vi "ДЗ Файлы.vi"() -> ()   [LabVIEW 2021]
panel:
  out "text":string
  out "XY Graph":cluster{i32[], dbl[]}[](graph)
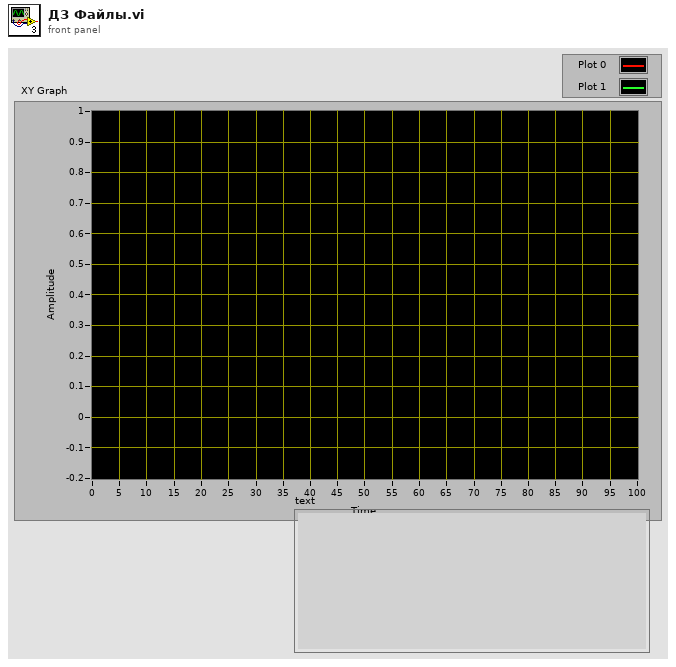
[diagram p1: front panel]
types:
  T1 = enum16{"open", "replace", "create", "open or create", "replace or create", "replace or create with confirmation"}
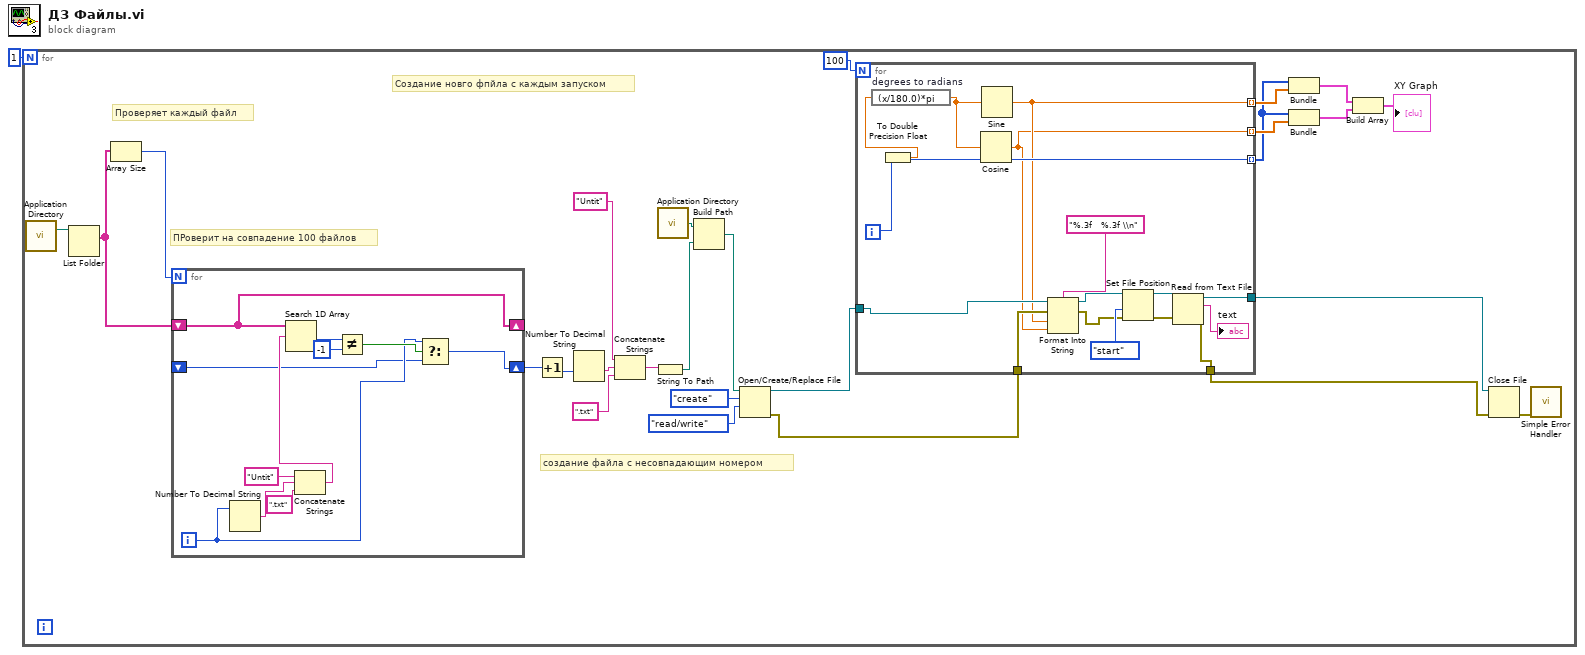
[diagram p0: block diagram]
diagram:
  n1 = for {
    N: 1 -> [_]
    # "Проверяет каждый файл"
    # "создание файла с несовпадающим номером"
    # "ПРоверит на совпадение 100 файлов"
    # "Создание новго фпйла с каждым запуском"
    n2 = call <vilib>:"Application Directory.vi"() -> ("Application Directory"=w18:path)
    n3 = List Folder(path=w18) -> (filenames=w2:string[])  [unwired: 3 in, 3 out]
    n4 = Array Size(array=w2) -> (size(s)=w3:i32)
    n5 = for {
      N: w3 -> [_]
      shift-right: [w48] -> _
      shift-left: w2 -> [w48]
      shift-right: [w44] -> w17
      shift-left: _ -> [w45]
      i -> [w46]
      n6 = Number To Decimal String(number=w46) -> (decimal integer string=w52:string)  [unwired: 1 in]
      n7 = Concatenate Strings("Untit" ("string"), w52, ".txt" ("string")) -> (w51:string)
      n8 = Search 1D Array(1D array=w48, element=w51) -> (index of element=w50:i32)  [unwired: 1 in]
      n9 = Not Equal?(x=w50, y=-1) -> (x != y?=w47:bool)
      n10 = Select(t=w46, s=w47, f=w45) -> (s? t:f=w44:i32)
    }
    n11 = Increment(x=w17) -> (x+1=w16:i32)
    n12 = Number To Decimal String(number=w16) -> (decimal integer string=w15:string)  [unwired: 1 in]
    n13 = Concatenate Strings("Untit" ("string"), w15, ".txt" ("string")) -> (w21:string)
    n14 = String To Path(string=w21) -> (path=w22:path)
    n15 = call <vilib>:"Application Directory.vi"() -> ("Application Directory"=w23:path)
    n16 = Build Path(base path=w23, name or relative path=w22) -> (appended path=w24:path)
    n17 = Open/Create/Replace File(file path (use dialog)=w24, operation (0:open)=T1."create", access (0:read/write)=enum16{"read/write", "read-only", "write-only"}."read/write") -> (refnum out=w7:refnum<file>, error out=w6:errorcluster)  [unwired: 3 in, 1 out]
    n18 = for {
      N: 100 -> [_]
      tunnel: [w29] -> w10 mode=indexing
      tunnel: [w28] -> w14 mode=indexing
      tunnel: [w36] -> w8 mode=indexing
      tunnel: w7 -> [w30]
      tunnel: w6 -> [w31]
      tunnel: [w39] -> w5
      tunnel: [w38] -> w4
      i -> [w36]
      n19 = To Double Precision Float(number=w36) -> (double precision float=w43:dbl)
      n20 = expression code="(x/180.0)*pi" "degrees to radians"(w43) -> (w35:dbl)
      n21 = Cosine(x=w35) -> (cos(x)=w28:dbl)
      n22 = Sine(x=w35) -> (sin(x)=w29:dbl)
      n23 = Format Into String(format string="%.3f   %.3f \\n", initial string=w30, error in=w31, w29, w28) -> (resulting string=w33:refnum<file>, error out=w32:errorcluster)
      n24 = Set File Position(refnum=w33, from (0:start)=enum16{"start", "end", "current"}."start", error in=w32) -> (refnum out=w40:refnum<file>, error out=w41:errorcluster)  [unwired: 1 in]
      n25 = Read from Text File(file (use dialog)=w40, error in=w41) -> (refnum out=w38:refnum<file>, text=→"text":string, error out=w39:errorcluster)  [unwired: 2 in, 1 out]
    }
    n26 = Bundle(w8, w10) -> (w9:cluster{i32[], dbl[]})  [unwired: 1 in]
    n27 = Bundle(w8, w14) -> (w13:cluster{i32[], dbl[]})  [unwired: 1 in]
    n28 = Build Array(w9, w13) -> (→"XY Graph":cluster{i32[], dbl[]}[])
    n29 = Close File(refnum=w4, error in=w5) -> (error out=w25:errorcluster)  [unwired: 1 out]
    n30 = call <vilib>:"Simple Error Handler.vi"("error in (no error)"=w25) -> ()  [unwired: 4 in, 5 out]
  }
